vi "Select Memory Location.vi"(8 "error in (no error)":errorcluster, 9 "Memory Location":u32 max=99 step=1, 10 "Memory":u32(ring) items=["Not Available", "Available"], 11 "VISA resource name":refnum<visa-resource-name>="TCPIP0::192.168.0.200::50505::SOCKET") -> (0 "error out":errorcluster, 3 "VISA resource name out":refnum<visa-resource-name>="TCPIP0::192.168.0.200::50505::SOCKET")   [LabVIEW 2022 SP3, in "MagnaDC.lvlib"]
uses:
  MagnaDC.lvlib
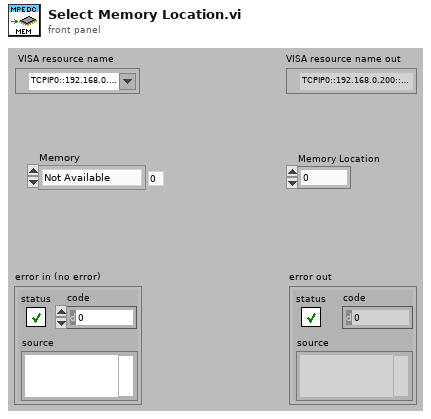
[diagram p1: front panel]
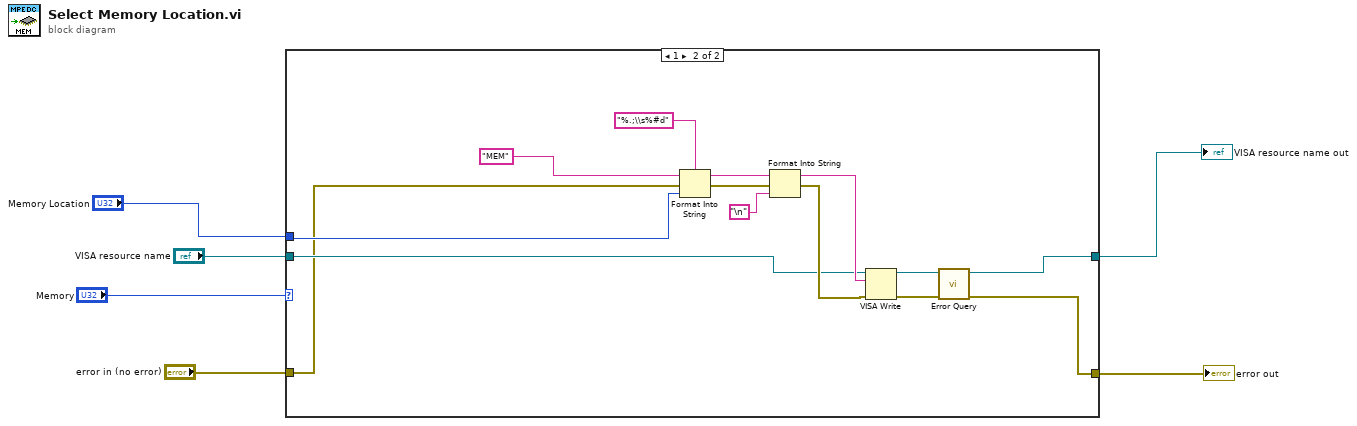
[diagram p0: block diagram]
diagram:
  n1 = case shown="1" "Memory" {
    tunnel: "VISA resource name" -> [w8 w12]
    tunnel: [w8 w11] -> w4
    tunnel: "error in (no error)" -> [w7 w9]
    tunnel: "Memory Location" -> [_ w13]
    tunnel: [w7 w10] -> w1
    frame 0, Default {
    }
    frame 1 {
      n2 = Format Into String(format string="%.;\\s%#d", initial string="MEM", error in=w9, w13) -> (resulting string=w22:string, error out=w21:errorcluster)
      n3 = Format Into String(initial string=w22, error in=w21, "\n") -> (resulting string=w19:string, error out=w20:errorcluster)  [unwired: 1 in]
      n4 = VISA Write(VISA resource name=w12, write buffer=w19, error in (no error)=w20) -> (VISA resource name out=w17:refnum<visa-resource-name>, error out=w18:errorcluster)  [unwired: 1 out]
      n5 = call "Error Query.vi"("error in (no error)"=w18, "VISA resource name"=w17) -> ("error out"=w10:errorcluster, "VISA resource name out"=w11:refnum<visa-resource-name>)  [unwired: 6 in, 2 out]
    }
  }
  "error out" <- w1
  "VISA resource name out" <- w4
